vi "Write Add Container Name to Tag.vi"(8 "error in (no error)":errorcluster, 10 "Add Container Name to Tag":bool, 11 "SharedVariable_Bus in":refnum<class "SharedVariable_Bus.lvclass">) -> (0 "error out":errorcluster, 3 "SharedVariable_Bus out":refnum<class "SharedVariable_Bus.lvclass">)   [LabVIEW 2021, in "SharedVariable_Bus.lvclass"]
uses:
  SharedVariable_Bus.lvclass
  SharedVariable_Bus.lvclass/SharedVariable_Bus.ctl
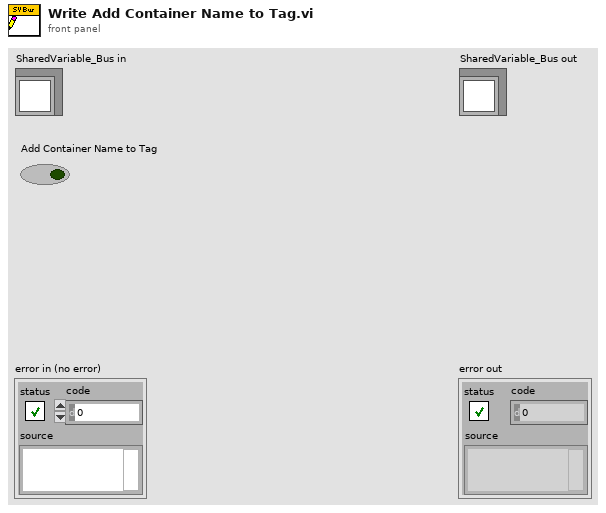
[diagram p1: front panel]
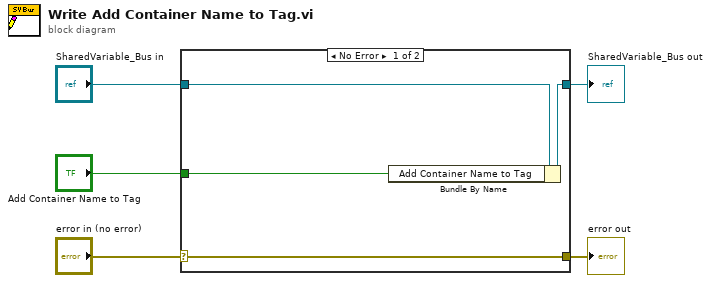
[diagram p0: block diagram]
diagram:
  n1 = case shown="No Error" "error in (no error)" {
    selector: "error in (no error)" -> [w9 w10]
    tunnel: [w9 w10] -> w4
    tunnel: [w7 w11] -> w2
    tunnel: "SharedVariable_Bus in" -> [w8 w11]
    tunnel: "Add Container Name to Tag" -> [w6 _]
    frame No Error {
      n2 = Bundle By Name(cluster=w8, "Add Container Name to Tag"=w6) -> (w7:refnum<class "SharedVariable_Bus.lvclass">)
    }
    frame Error {
    }
  }
  "error out" <- w4
  "SharedVariable_Bus out" <- w2
